vi "Key_Init.vi"(3 "Container State":T3 caption="牧抛捞呈 惑怕", 4 "Previous State":variant caption="捞傈 惑怕", 5 "Previous Version":T2 caption="捞傈 滚傈") -> (2 "Current State":T1 caption="泅犁 惑怕")   [LabVIEW 2012, in "Key_Xcontrol.xctl"]
uses:
  Key_Xcontrol.xctl
  Key_State.ctl
  <vilib>/_xctls/Container State.ctl
  <vilib>/_xctls/Version.ctl
  <vilib>/_xctls/XControlSupport.lvlib
panel:
  in  "Default Indicator State":T1 caption="扁夯 牢叼纳捞磐 惑怕"
  in  "Default Control State":T1 caption="扁夯 牧飘费 惑怕"
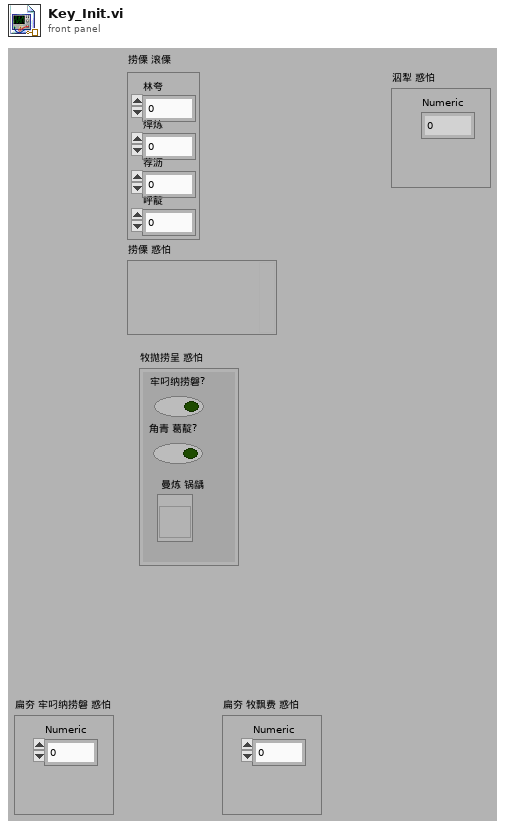
[diagram p1: front panel]
types:
  T1 = typedef "Key_Xcontrol.xctl/Key_State.ctl" = cluster{"Numeric":u8}
  T2 = typedef "XControlSupport.lvlib/Version.ctl" = cluster{"Major":u16, "Minor":u16, "Fix":u16, "Build":u16}
  T3 = typedef "XControlSupport.lvlib/Container State.ctl" = cluster{"Indicator?":bool, "Run Mode?":bool, " Refnum":refnum<vi>}
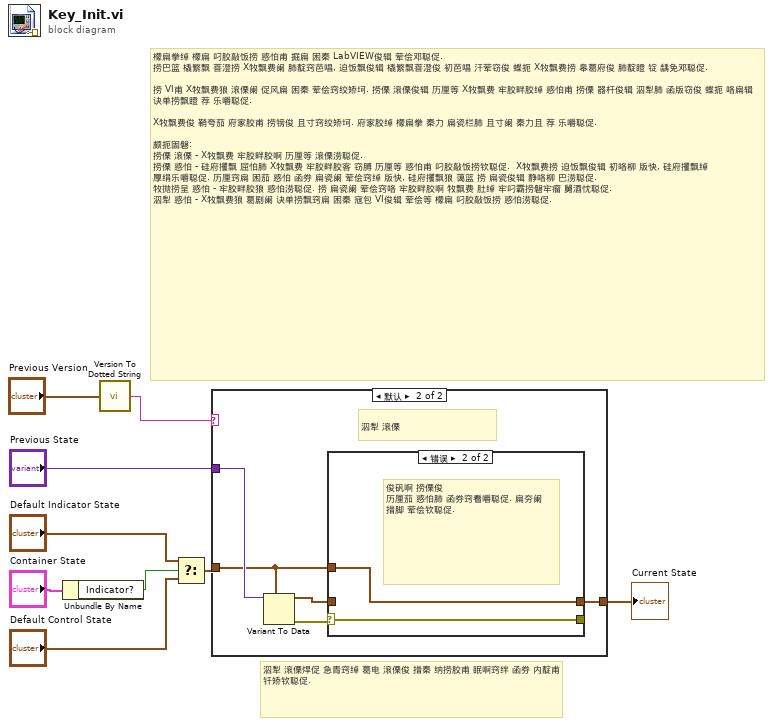
[diagram p0: block diagram]
diagram:
  # "泅犁 滚傈焊促 急青窍绰 葛电 滚傈俊 措秦 纳捞胶甫 眠啊窍绊 函券 内靛甫 钎矫钦聪促."
  # "檬扁拳绰 檬扁 叼胶敲饭捞 惑怕甫 掘扁 困秦 LabVIEW俊辑 荤侩邓聪促.\n捞巴篮 橇繁飘 菩澄捞 X牧飘费阑 肺靛窍芭唱, 迫饭飘俊辑 橇繁飘菩澄俊 初芭唱 汗荤窃俊 蝶扼 X牧飘费捞 皋葛府俊 肺靛瞪 锭 龋免邓聪促.\n\n捞 VI甫 X牧飘费狼 滚傈阑 促风扁 困秦 荤侩窍绞矫坷. 捞傈 滚傈俊辑 历厘等 X牧飘费 牢胶畔胶绰 惑怕甫 捞傈 器杆俊辑 泅犁肺 函版窃俊 蝶扼 咯扁辑 诀单捞飘瞪 荐 乐嚼聪促.\n\nX牧飘费俊 鞘夸茄 府家胶甫 捞镑俊 且寸窍绞矫坷. 府家胶绰 檬扁拳 秦力 扁瓷栏肺 且寸阑 秦力且 荐 乐嚼聪促.\n\n颇扼固磐:\n捞傈 滚傈 - X牧飘费 牢胶畔胶啊 历厘等 滚傈涝聪促.\n捞傈 惑怕 - 硅府攫飘 屈怕肺 X牧飘费 牢胶畔胶客 窃膊 历厘等 惑怕甫 叼胶敲饭捞钦聪促.  X牧飘费捞 迫饭飘俊辑 初咯柳 版快, 硅府攫飘绰 厚绢乐嚼聪促. 历厘窍扁 困茄 惑怕 函券 扁瓷阑 荤侩窍绰 版快, 硅府攫飘狼 蔼篮 捞 扁瓷俊辑 静咯柳 巴涝聪促. \n牧抛捞呈 惑怕 - 牢胶畔胶狼 惑怕涝聪促. 捞 扁瓷阑 荤侩窍咯 牢胶畔胶啊 牧飘费 肚绰 牢叼霸捞磐牢瘤 舅酒忱聪促.\n泅犁 惑怕 - X牧飘费狼 葛剧阑 诀单捞飘窍扁 困秦 寇包 VI俊辑 荤侩等 檬扁 叼胶敲饭捞 惑怕涝聪促."
  n1 = Unbundle By Name("Container State") -> ("Indicator?"=w4:bool)
  n2 = call <vilib>:"Version To Dotted String.vi"("Version"="Previous Version") -> ("String Version"=w1:string)
  n3 = Select(t="Default Indicator State", s=w4, f="Default Control State") -> (s? t:f=w3:T1)
  n4 = case shown="默认" w1 {
    tunnel: "Previous State" -> [_ w15]
    tunnel: [w10 w11] -> w8
    tunnel: w3 -> [w10 w12]
    frame "0.0.0.0" {
      # "规陛 积己凳, 扁夯 惑怕 荤侩"
    }
    frame Default {
      # "泅犁 滚傈"
      n5 = Variant To Data(type=w12, Variant=w15) -> (data=w13:T1, error out=w14:errorcluster)  [unwired: 1 in]
      n6 = case shown="错误" w14 {
        selector: w14 -> [w17 w18]
        tunnel: w13 -> [w16 _]
        tunnel: [w16 w19] -> w11
        tunnel: w12 -> [_ w19]
        tunnel: [w17 w18] -> _
        frame No Error {
        }
        frame Error {
          # "俊矾啊 捞傈俊\n历厘茄 惑怕肺 函券窍看嚼聪促. 扁夯阑 措脚 荤侩钦聪促."
        }
      }
    }
  }
  "Current State" <- w8
